vi "ForceAngleTo_0_360.vi"(8 "error in (no error)":errorcluster, 11 "Angle in":refnum<class "Angle.lvclass">) -> (0 "error out":errorcluster, 2 "Relative Angle":dbl)   [LabVIEW 2013, in "Angle.lvclass"]
doc: "Takes in an angle object between -360 and 720, outputs the angle as a double, in between 0-360.\n\nEric Schneider, Feb. 2014"
uses:
  Angle.lvclass
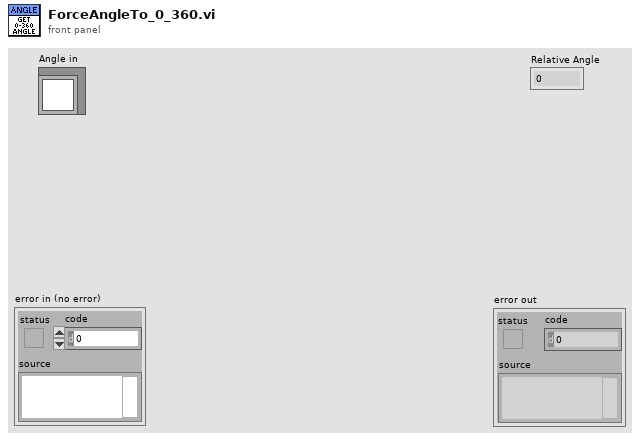
[diagram p1: front panel]
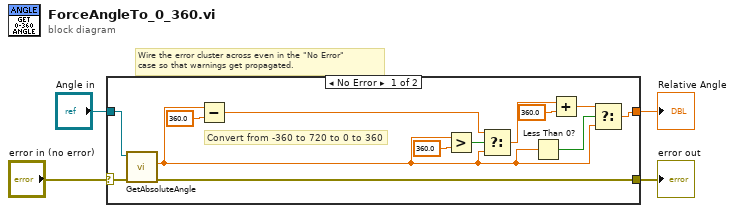
[diagram p0: block diagram]
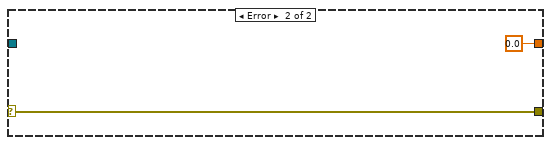
[diagram p2: hidden frame]
diagram:
  # "Wire the error cluster across even in the \"No Error\"\ncase so that warnings get propagated."
  n1 = case shown="No Error" "error in (no error)" {
    selector: "error in (no error)" -> [w12 w19]
    tunnel: [w11 w19] -> w3
    tunnel: "Angle in" -> [w13 _]
    tunnel: [w5 0.0 ("New Angle")] -> w1
    frame No Error {
      # "Convert from -360 to 720 to 0 to 360"
      n2 = call "GetAbsoluteAngle.vi"("error in (no error)"=w12, "Angle in"=w13) -> ("error out"=w11:errorcluster, "Absolute angle (Deg.)"=w9:dbl)  [unwired: 8 in]
      n3 = Subtract(x=w9, y=360.0) -> (x-y=w15:dbl)
      n4 = Greater?(x=w9, y=360.0) -> (0:w17:bool)
      n5 = Select(t=w15, s=w17, f=w9) -> (s? t:f=w6:dbl)
      n6 = Less Than 0?(x=w9) -> (x < 0?=w10:bool)
      n7 = Add(x=w6, y=360.0) -> (x+y=w7:dbl)
      n8 = Select(t=w7, s=w10, f=w9) -> (s? t:f=w5:dbl)
    }
    frame Error {
    }
  }
  "error out" <- w3
  "Relative Angle" <- w1
